vi "serial_control_test.vi"() -> ()   [LabVIEW 2014]
uses:
  <vilib>/Instr/_visa.llb/VISA Configure Serial Port (Instr).vi
panel:
  in  "Ethernal COM Port":refnum<visa-resource-name>="COM1"
  in  "Controller Stop":bool
  in  "Control Rate (ms)":u32=290
  out "Hardware Enabled":bool=TRUE
  out "Software Enabled":bool=TRUE
  out "Temp Stable":bool=TRUE
  in  "Which Temp?":enum16{"ETH", "PUMP", "PCB", "AMP", "CASE"}(ring)
  out "Temp":i32(graph)
  out "Power":i32(graph)
  in  "Change Power?":bool=TRUE
  in  "LEVEL CONTROL, 0-100 (%)":u8(knob) scale=0.0..100.0
  in  "ENABLE":bool
  in  "DISABLE":bool
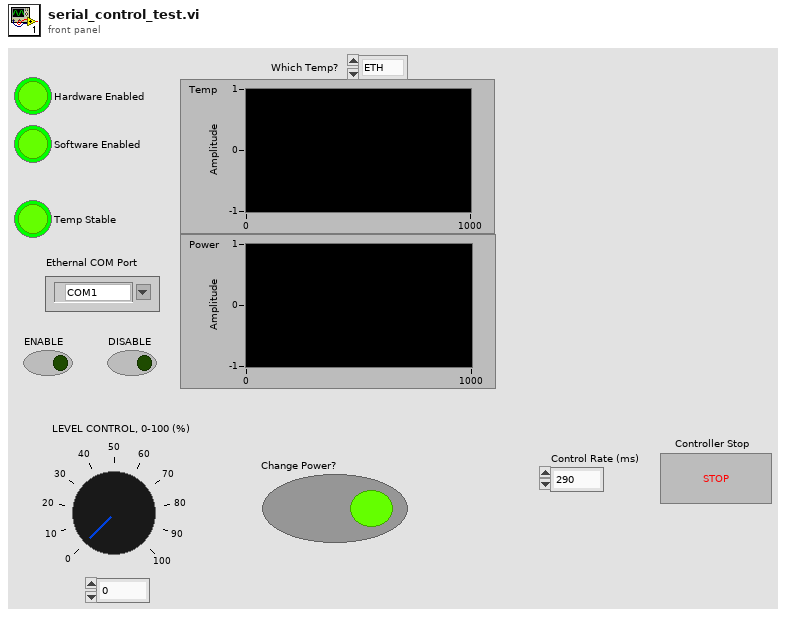
[diagram p1: front panel]
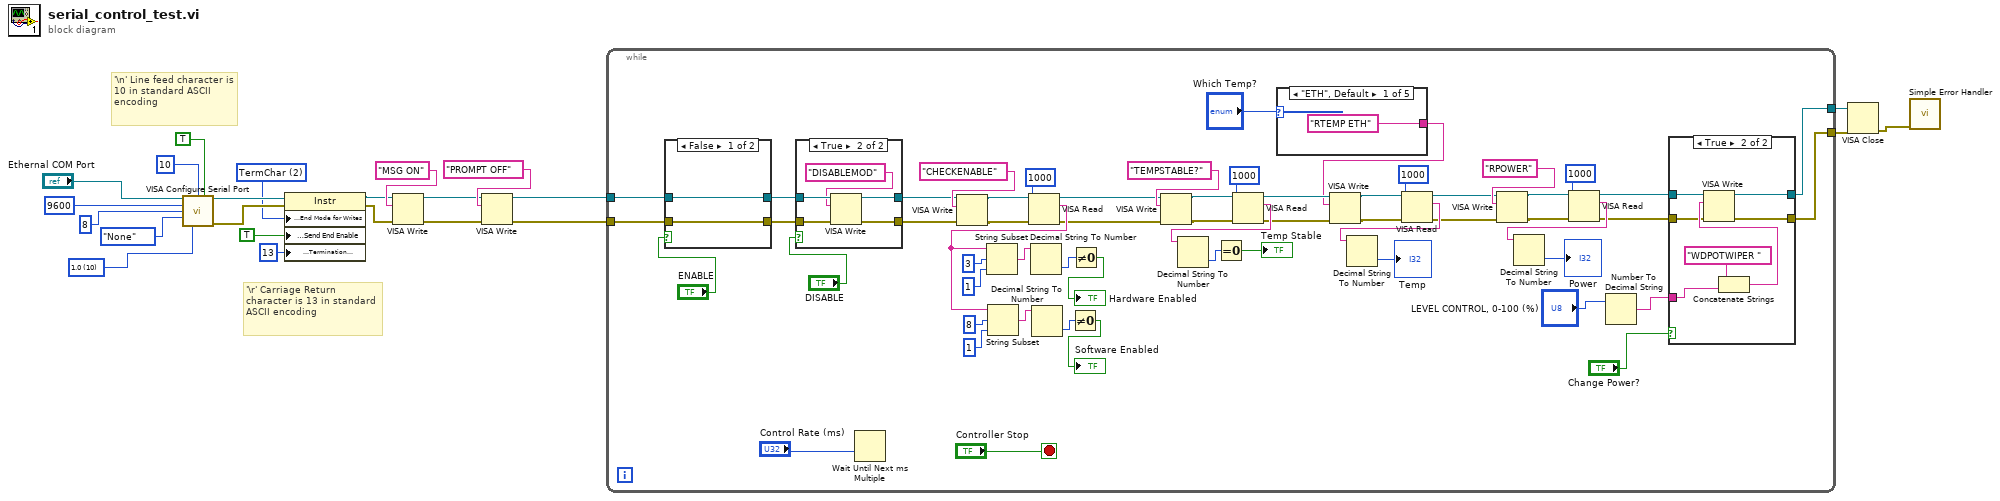
[diagram p0: block diagram]
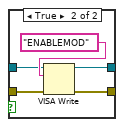
[diagram p3: hidden frame]
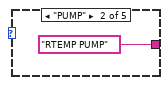
[diagram p5: hidden frame]
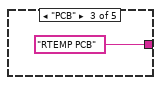
[diagram p6: hidden frame]
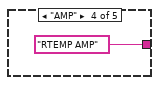
[diagram p7: hidden frame]
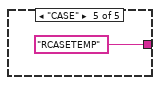
[diagram p8: hidden frame]
diagram:
  w6 = u16 10 items=["1.0"=10, "1.5"=15, "2.0"=20] ("stop bits (10: 1 bit)")
  w20 = u16 2 items=["None", "LastBit", "TermChar", "Break"] ("Serial Settings:Serial End Mode for Writes")
  # "'\\r' Carriage Return character is 13 in standard ASCII encoding"
  # "'\\n' Line feed character is 10 in standard ASCII encoding"
  n1 = call-poly "VISA Configure Serial Port"("VISA resource name"="Ethernal COM Port", "termination char\n(0xA = '\\n' = LF)"=u8 10, "Enable Termination\nChar (T)"=TRUE, "baud rate (9600)"=u32 9600, "data bits (8)"=u16 8, "parity (0:none)"=enum16{"None", "Odd", "Even", "Mark", "Space"}."None", "stop bits (10: 1 bit)"=w6) -> ("VISA resource name out"=w22:refnum<visa-resource-name>, "error out"=w23:errorcluster)  [unwired: 3 in, 4 out]
  n2 = property class="Instr"(reference=w22, error in=w23, "Serial Settings:End Mode for Writes"=w20, "Message Based Settings:Send End Enable"=TRUE, "Message Based Settings:Termination Character"=13) -> (reference out=w11:refnum<visa-resource-name>, error out=w12:errorcluster)
  n3 = VISA Write(VISA resource name=w11, write buffer="MSG ON" ("Enable 2"), error in (no error)=w12) -> (VISA resource name out=w9:refnum<visa-resource-name>, error out=w8:errorcluster)  [unwired: 1 out]
  n4 = VISA Write(VISA resource name=w9, write buffer="PROMPT OFF" ("Enable 2"), error in (no error)=w8) -> (VISA resource name out=w5:refnum<visa-resource-name>, error out=w4:errorcluster)  [unwired: 1 out]
  n5 = while {
    tunnel: [w33] -> w3
    tunnel: [w32] -> w2
    tunnel: w5 -> [w25]
    tunnel: w4 -> [w24]
    stop <- "Controller Stop" stop-if-true
    n6 = case shown="False" "ENABLE" {
      tunnel: [w90 w95] -> w31
      tunnel: [w89 w94] -> w30
      tunnel: w25 -> [w90 w92]
      tunnel: w24 -> [w89 w91]
      frame False {
      }
      frame True {
        n7 = VISA Write(VISA resource name=w92, write buffer="ENABLEMOD" ("Enable 2"), error in (no error)=w91) -> (VISA resource name out=w95:refnum<visa-resource-name>, error out=w94:errorcluster)  [unwired: 1 out]
      }
    }
    n8 = case shown="True" "DISABLE" {
      tunnel: w31 -> [w83 w88]
      tunnel: w30 -> [w82 w87]
      tunnel: [w83 w86] -> w29
      tunnel: [w82 w85] -> w28
      frame False {
      }
      frame True {
        n9 = VISA Write(VISA resource name=w88, write buffer="DISABLEMOD" ("Enable 2"), error in (no error)=w87) -> (VISA resource name out=w86:refnum<visa-resource-name>, error out=w85:errorcluster)  [unwired: 1 out]
      }
    }
    n10 = Wait Until Next ms Multiple(millisecond multiple="Control Rate (ms)") -> ()  [unwired: 1 out]
    n11 = VISA Write(VISA resource name=w29, write buffer="CHECKENABLE" ("Enable 2"), error in (no error)=w28) -> (VISA resource name out=w77:refnum<visa-resource-name>, error out=w76:errorcluster)  [unwired: 1 out]
    n12 = VISA Read(VISA resource name=w77, byte count=u32 1000 ("Read Count"), error in (no error)=w76) -> (VISA resource name out=w59:refnum<visa-resource-name>, read buffer=w71:string, error out=w58:errorcluster)  [unwired: 1 out]
    n13 = String Subset(string=w71, offset (0)=3, length (rest)=1) -> (substring=w70:string)
    n14 = String Subset(string=w71, offset (0)=8, length (rest)=1) -> (substring=w69:string)
    n15 = Decimal String To Number(string=w70) -> (number=w68:i32)  [unwired: 2 in, 1 out]
    n16 = Decimal String To Number(string=w69) -> (number=w65:i32)  [unwired: 2 in, 1 out]
    n17 = Not Equal To 0?(x=w65) -> (x != 0?=→"Software Enabled":bool)
    n18 = Not Equal To 0?(x=w68) -> (x != 0?=→"Hardware Enabled":bool)
    n19 = VISA Write(VISA resource name=w59, write buffer="TEMPSTABLE?" ("Enable 2"), error in (no error)=w58) -> (VISA resource name out=w62:refnum<visa-resource-name>, error out=w61:errorcluster)  [unwired: 1 out]
    n20 = VISA Read(VISA resource name=w62, byte count=u32 1000 ("Read Count 3"), error in (no error)=w61) -> (VISA resource name out=w51:refnum<visa-resource-name>, read buffer=w60:string, error out=w50:errorcluster)  [unwired: 1 out]
    n21 = Decimal String To Number(string=w60) -> (number=w56:i32)  [unwired: 2 in, 1 out]
    n22 = Equal To 0?(x=w56) -> (x = 0?=→"Temp Stable":bool)
    n23 = case shown="\"ETH\", Default" "Which Temp?" {
      tunnel: ["RTEMP ETH" ("Enable 2") "RTEMP PUMP" ("Enable 2") "RTEMP PCB" ("Enable 2") "RTEMP AMP" ("Enable 2") "RCASETEMP" ("Enable 2")] -> w49
      frame "ETH", Default {
      }
      frame "PUMP" {
      }
      frame "PCB" {
      }
      frame "AMP" {
      }
      frame "CASE" {
      }
    }
    n24 = VISA Write(VISA resource name=w51, write buffer=w49, error in (no error)=w50) -> (VISA resource name out=w53:refnum<visa-resource-name>, error out=w52:errorcluster)  [unwired: 1 out]
    n25 = VISA Read(VISA resource name=w53, byte count=u32 1000 ("Read Count 3"), error in (no error)=w52) -> (VISA resource name out=w42:refnum<visa-resource-name>, read buffer=w48:string, error out=w41:errorcluster)  [unwired: 1 out]
    n26 = Decimal String To Number(string=w48) -> (number=→"Temp":i32)  [unwired: 2 in, 1 out]
    n27 = VISA Write(VISA resource name=w42, write buffer="RPOWER" ("Enable 2"), error in (no error)=w41) -> (VISA resource name out=w45:refnum<visa-resource-name>, error out=w44:errorcluster)  [unwired: 1 out]
    n28 = VISA Read(VISA resource name=w45, byte count=u32 1000 ("Read Count 3"), error in (no error)=w44) -> (VISA resource name out=w35:refnum<visa-resource-name>, read buffer=w40:string, error out=w34:errorcluster)  [unwired: 1 out]
    n29 = Decimal String To Number(string=w40) -> (number=→"Power":i32)  [unwired: 2 in, 1 out]
    n30 = Number To Decimal String(number="LEVEL CONTROL, 0-100 (%)") -> (decimal integer string=w36:string)  [unwired: 1 in]
    n31 = case shown="True" "Change Power?" {
      tunnel: w36 -> [_ w103]
      tunnel: w35 -> [w97 w101]
      tunnel: w34 -> [w96 w100]
      tunnel: [w97 w99] -> w33
      tunnel: [w96 w98] -> w32
      frame False {
      }
      frame True {
        n32 = Concatenate Strings("WDPOTWIPER " ("Enable 2"), w103) -> (w102:string)
        n33 = VISA Write(VISA resource name=w101, write buffer=w102, error in (no error)=w100) -> (VISA resource name out=w99:refnum<visa-resource-name>, error out=w98:errorcluster)  [unwired: 1 out]
      }
    }
  }
  n34 = VISA Close(VISA resource name=w3, error in (no error)=w2) -> (error out=w1:errorcluster)
  n35 = call <vilib>:"Simple Error Handler.vi"("error in (no error)"=w1) -> ()  [unwired: 4 in, 5 out]
